vi "sub_SDR_mod_BPSK_To_4QAM.vi"(11 "Array in":i16[](array[numeric])) -> (3 "Array out":cdb[](array[numeric]))   [LabVIEW 2012]
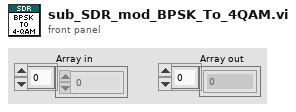
[diagram p1: front panel]
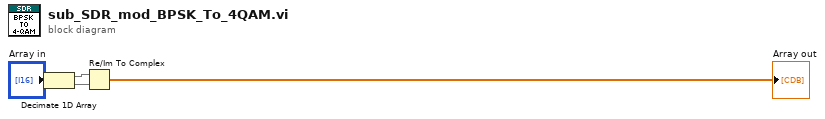
[diagram p0: block diagram]
diagram:
  n1 = Decimate 1D Array("Array in") -> (w1:i16[], w2:i16[])
  n2 = Re/Im To Complex(1:w2, 2:w1) -> (0:→"Array out":cdb[])
